vi "CRYTree Selection Reorder.vi"(7 "sAction":string="GetActiveSymbols", 10 "Symbol In":i32[](array[numeric]), 11 "Number In":i32[](array[numeric])) -> (2 "Symbol Out":i32[](array[numeric]), 3 "Number Out":i32[](array[numeric]))   [LabVIEW 2013]
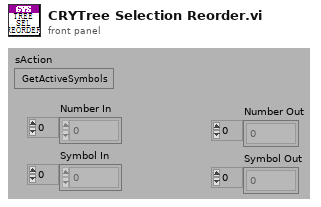
[diagram p1: front panel]
types:
  T1 = cluster{"nData 2":i32, "Active Item Row Number":i32}
  T2 = cluster{"nData 2":i32, "Active Item Row Number":i32}[]
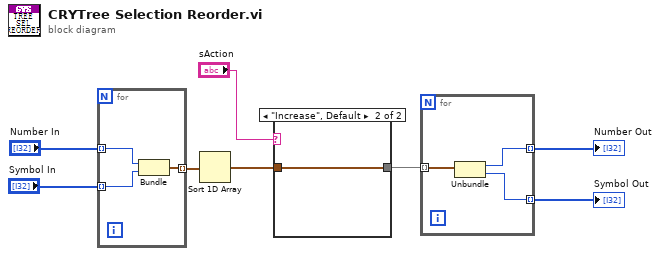
[diagram p0: block diagram]
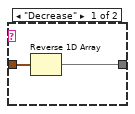
[diagram p2: hidden frame]
diagram:
  n1 = for {
    tunnel: "Number In" -> [w11] mode=indexing
    tunnel: "Symbol In" -> [w10] mode=indexing
    tunnel: [w9] -> w6 mode=indexing
    n2 = Bundle("nData 2"=w11, "Active Item Row Number"=w10) -> (w9:T1)  [unwired: 1 in]
  }
  n3 = Sort 1D Array(array=w6) -> (sorted array=w3:T2)
  n4 = case shown="\"Increase\", Default" "sAction" {
    tunnel: w3 -> [w13 w14]
    tunnel: [w12 w14] -> w2
    frame "Decrease" {
      n5 = Reverse 1D Array(array=w13) -> (reversed array=w12:T2)
    }
    frame "Increase", Default {
    }
  }
  n6 = for {
    tunnel: w2 -> [w17] mode=indexing
    tunnel: [w16] -> w5 mode=indexing
    tunnel: [w15] -> w4 mode=indexing
    n7 = Unbundle(w17) -> ("nData 2"=w16:i32, "Active Item Row Number"=w15:i32)
  }
  "Symbol Out" <- w4
  "Number Out" <- w5
